vi "applyPresetAllChannels.vi"(8 "error in (no error)":errorcluster, 11 "DistanceGauge in":refnum<class "DistanceGauge.lvclass">) -> (0 "error out":errorcluster, 3 "DistanceGauge out":refnum<class "DistanceGauge.lvclass">)   [LabVIEW 2015, in "DistanceGauge.lvlib" / "DistanceGauge.lvclass"]
uses:
  <userlib>/Common/Devices/DistanceGauge/DistanceGauge/DistanceGauge.lvclass
  <userlib>/Common/Devices/DistanceGauge/DistanceGauge/DistanceGauge.lvclass/DistanceGauge.ctl
  <userlib>/Common/SerialProtocols/SerialCommunicator/SerialCommunicator.lvclass
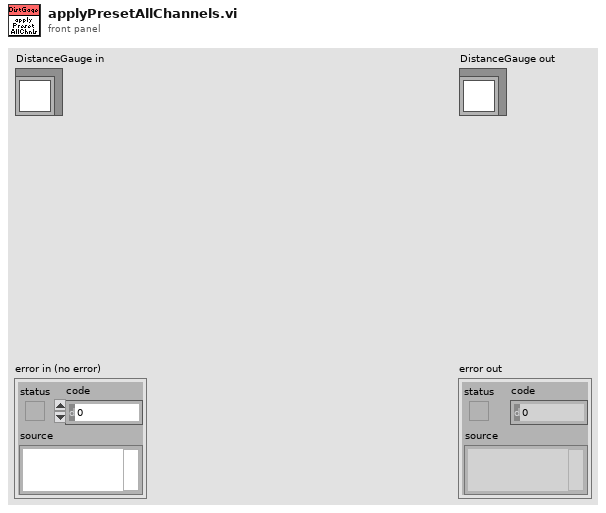
[diagram p1: front panel]
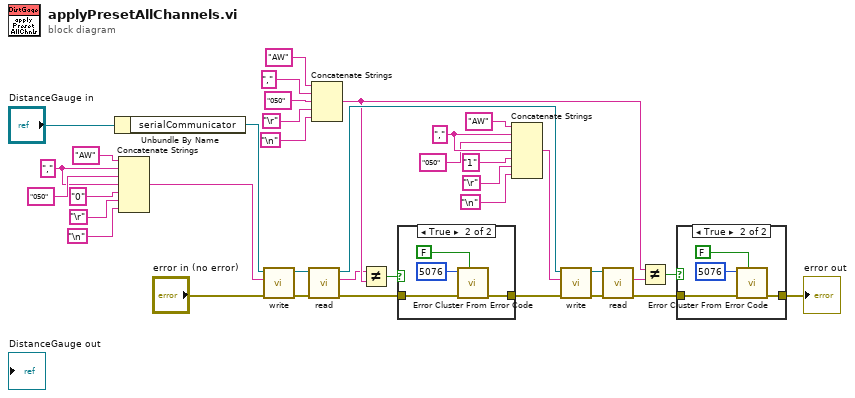
[diagram p0: block diagram]
diagram:
  w20 = "," ("writeString")
  w26 = "," ("writeString")
  n1 = Unbundle By Name("DistanceGauge in") -> ("serialCommunicator"=w36:refnum<class "SerialCommunicator.lvclass">)
  n2 = Concatenate Strings("AW" ("writeString"), w26, "050" ("string"), w26, "0" ("string"), "\r", "\n") -> (w31:string)
  n3 = call-dynamic "write.vi"("error in (no error)"="error in (no error)", "writeString"=w31, "SerialCommunicator in"=w36) -> ("error out"=w33:errorcluster, "SerialCommunicator out"=w35:refnum<class "SerialCommunicator.lvclass">)  [unwired: 7 in]
  n4 = call-dynamic "read.vi"("error in (no error)"=w33, "SerialCommunicator in"=w35) -> ("error out"=w8:errorcluster, "stringRead"=w4:string, "SerialCommunicator out"=w22:refnum<class "SerialCommunicator.lvclass">)  [unwired: 7 in]
  n5 = Concatenate Strings("AW" ("writeString"), "," ("writeString"), "050" ("string"), "\r", "\n") -> (w5:string)
  n6 = Not Equal?(x=w4, y=w5) -> (x != y?=w9:bool)
  n7 = case shown="True" w9 {
    tunnel: w8 -> [w37 w40]
    tunnel: [w37 w39] -> w7
    frame False {
    }
    frame True {
      n8 = call <vilib>:"Error Cluster From Error Code.vi"("show call chain? (False)"=FALSE, "error in (no error)"=w40, "error code (0)"=5076) -> ("error out"=w39:errorcluster)  [unwired: 6 in]
    }
  }
  n9 = Concatenate Strings("AW" ("writeString"), w20, "050" ("string"), w20, "1" ("string"), "\r", "\n") -> (w15:string)
  n10 = call-dynamic "write.vi"("error in (no error)"=w7, "writeString"=w15, "SerialCommunicator in"=w22) -> ("error out"=w24:errorcluster, "SerialCommunicator out"=w23:refnum<class "SerialCommunicator.lvclass">)  [unwired: 7 in]
  n11 = call-dynamic "read.vi"("error in (no error)"=w24, "SerialCommunicator in"=w23) -> ("error out"=w2:errorcluster, "stringRead"=w3:string)  [unwired: 7 in, 1 out]
  n12 = Not Equal?(x=w5, y=w3) -> (x != y?=w6:bool)
  n13 = case shown="True" w6 {
    tunnel: w2 -> [w42 w45]
    tunnel: [w42 w43] -> w1
    frame False {
    }
    frame True {
      n14 = call <vilib>:"Error Cluster From Error Code.vi"("show call chain? (False)"=FALSE, "error in (no error)"=w45, "error code (0)"=5076) -> ("error out"=w43:errorcluster)  [unwired: 6 in]
    }
  }
  "error out" <- w1
